vi "driveStop.vi"() -> ()   [LabVIEW 2011]
uses:
  drivetrain/gear_shift_state.ctl
  drivetrain/drivetrain_drive_mode.ctl
  drivetrain/drivetrain_drive_write_thread.ctl
  drivetrain/drivetrain_globals.vi
panel:
  out "x > y?":bool
  in  "settle time":u32=250
  in  "stop deadband":dbl=1.5
  out "Waveform Chart":cluster{"Left":dbl, "Right":dbl}(graph)
  in  "max stop speed":dbl=1.5
  in  "kI":dbl=-0.008
  in  "kP":dbl=-0.1
  # "Old gains:\n\nkP -0.4\nkI -0.005\nmax stop speed 8\nstop deadband 1.5\nsettle time 250"
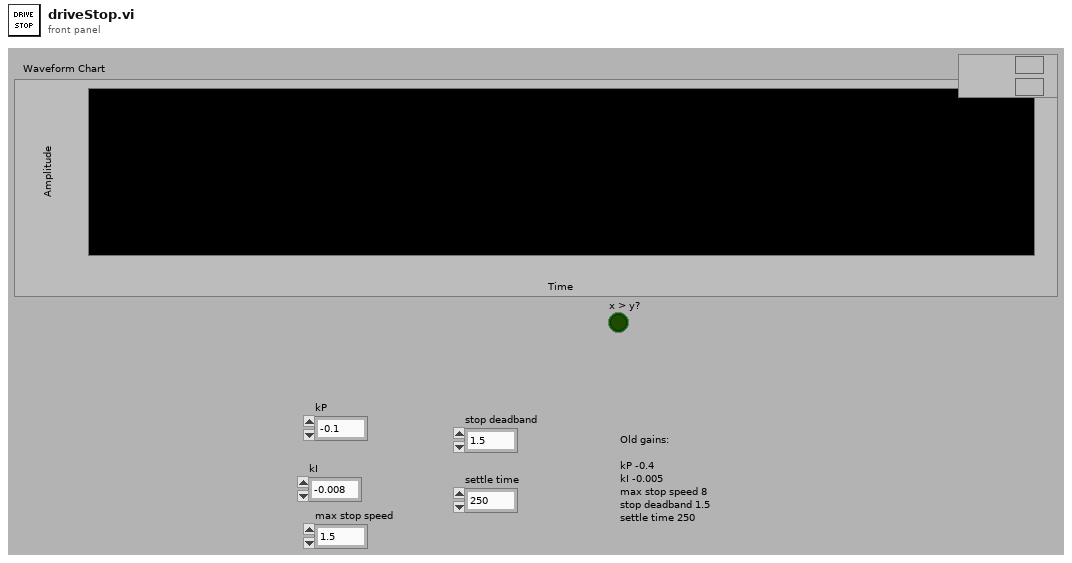
[diagram p1: front panel]
types:
  T1 = typedef "gear_shift_state.ctl" = enum16{"low", "high"}
  T2 = typedef "drivetrain_drive_mode.ctl" = enum16{"open loop", "closed loop"}
  T3 = typedef "drivetrain_drive_write_thread.ctl" = enum16{"Teleop", "Script Engine - Autonomous", "Script Engine - Sequence"}
  T4 = typedef "WPI_RobotDriveDevRef.ctl" = cluster{"DevStatus":errorcluster, "Motors[]":T5[], "Square Inputs":bool, "Max Output":dbl}
  T5 = typedef "WPI_MotorControlDeviceRef.ctl" = cluster{"DeviceStatus":errorcluster, "Type":enum16{"PWM", "CAN"}, "PWM":cluster{"Digital Module":T6, "PWM Channel":T7, "DeadBand":T8}, "CAN":cluster{"Device Number":u8, "Control Mode":T9, "Semaphore":T10, "Max Vout":dbl}, "Invert":bool, "TransformRef":T11, "InvTransformRef":T11}
  T6 = typedef "FPGA_TypedefDigitalModule.ctl" = enum16{"Digital Module 1", "Digital Module 2"}
  T7 = typedef "FPGA_DIOPWMChannel.ctl" = enum8{"PWM 1", "PWM 2", "PWM 3", "PWM 4", "PWM 5", "PWM 6", "PWM 7", "PWM 8", "PWM 9", "PWM 10", "Invalid"}
  T8 = typedef "WPI_PWMDeadband.ctl" = cluster{"Name":string, "maxPositivePwm":i32, "minPositivePwm":i32, "centerPwm":i32, "maxNegativePwm":i32, "minNegativePwm":i32, "angularRange":u16}
  T9 = typedef "WPI_CANJaguar_ControlMode.ctl" = enum8{"Percent VBus", "Current", "Speed", "Position", "Voltage"}
  T10 = typedef "Semaphore RefNum" = refnum<k1>
  T11 = typedef "WPI_PWMTransform_ConPane.ctl" = refnum<vi>
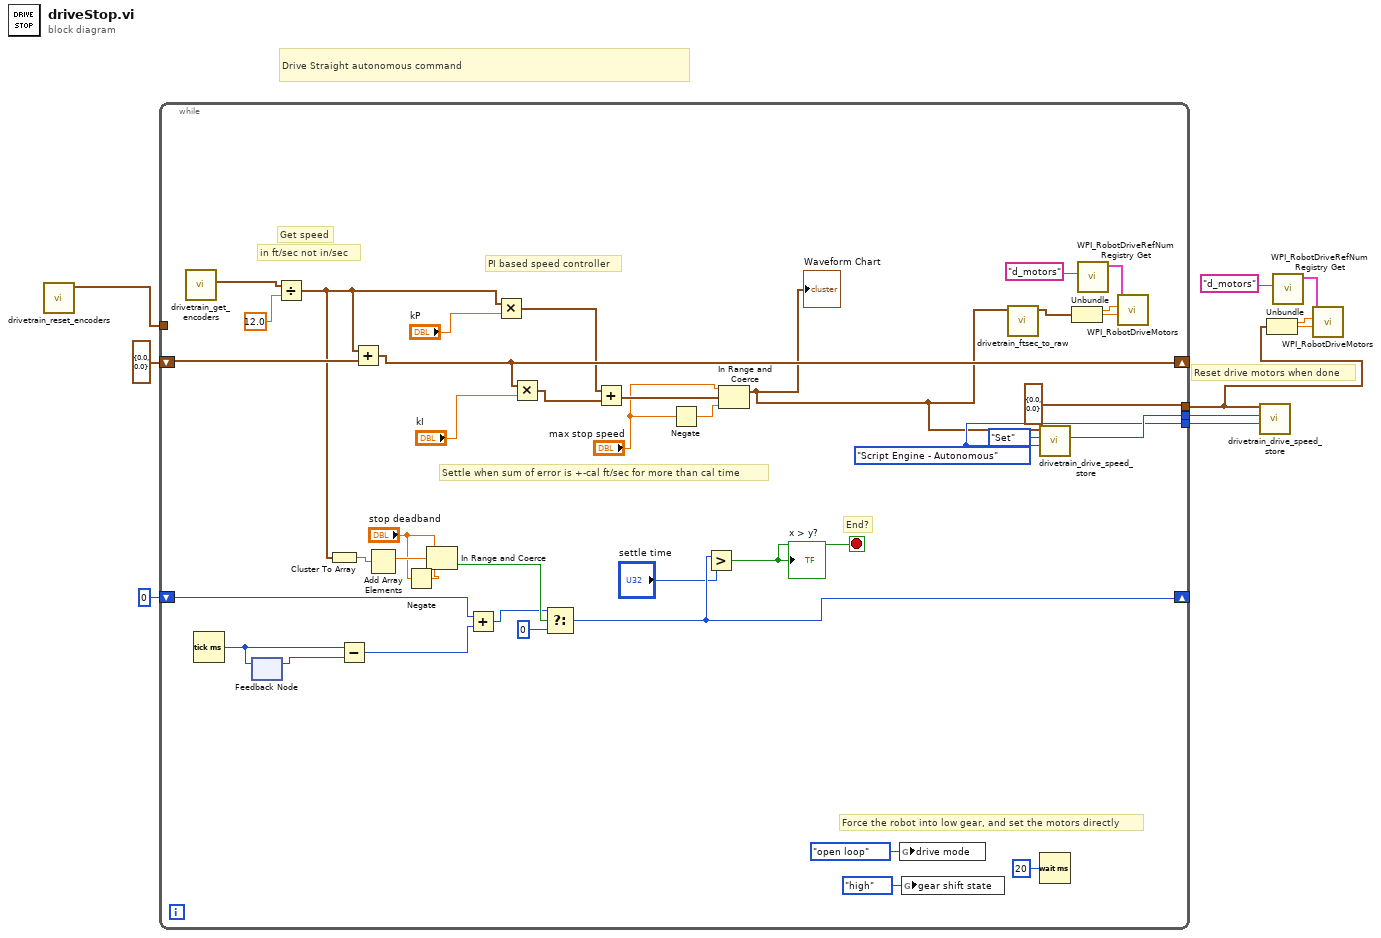
[diagram p0: block diagram]
diagram:
  # "Drive Straight autonomous command"
  # "Reset drive motors when done"
  n1 = call "drivetrain_reset_encoders.vi"() -> ("Distance (in)"=w10:cluster{"Left":dbl, "Right":dbl})  [unwired: 9 in, 2 out]
  n2 = while {
    tunnel: w10 -> [_]
    tunnel: [cluster{"Left":dbl, "Right":dbl} {"Left"=0.0, "Right"=0.0} ("Drive")] -> w5
    tunnel: [w46] -> w9
    tunnel: [w45] -> w8
    shift-right: [w33] -> _
    shift-left: cluster{"Left":dbl, "Right":dbl} {"Left"=0.0, "Right"=0.0} -> [w34]
    shift-right: [w14] -> _
    shift-left: u32 0 -> [w17]
    stop <- w11 stop-if-true
    w45 = drivetrain_drive_write_thread."Script Engine - Autonomous" ("Write Thread")
    w46 = enum16{"Set", "Get"}."Set" ("data_store_mode")
    # "Settle when sum of error is +-cal ft/sec for more than cal time"
    # "PI based speed controller"
    # "in ft/sec not in/sec"
    # "Get speed"
    # "End?"
    # "Force the robot into low gear, and set the motors directly"
    n3 = call "drivetrain_get_encoders.vi"() -> ("Velocity (in/sec)"=w37:cluster{"Left":dbl, "Right":dbl})  [unwired: 9 in, 2 out]
    n4 = Tick Count (ms)() -> (millisecond timer value=w20:u32)
    n5 = feedback-in #1(w20) -> ()
    n6 = feedback #1() -> (w19:u32)  [unwired: 1 in]
    n7 = Divide(x=w37, y=12.0) -> (x/y=w25:cluster{"Left":dbl, "Right":dbl})
    n8 = Cluster To Array(cluster=w25) -> (array=w24:dbl[])
    n9 = Subtract(x=w20, y=w19) -> (x-y=w12:u32)
    n10 = Add(x=w25, y=w34) -> (x+y=w33:cluster{"Left":dbl, "Right":dbl})
    n11 = Add Array Elements(numeric array=w24) -> (sum=w23:dbl)
    n12 = Negate(x="stop deadband") -> (-x=w22:dbl)
    n13 = In Range and Coerce(upper limit="stop deadband", x=w23, lower limit=w22) -> (In Range?=w18:bool)  [unwired: 1 out]
    n14 = Add(x=w17, y=w12) -> (x+y=w16:u32)
    n15 = Multiply(x=w25, y="kP") -> (x*y=w31:cluster{"Left":dbl, "Right":dbl})
    n16 = Multiply(x=w33, y="kI") -> (x*y=w30:cluster{"Left":dbl, "Right":dbl})
    n17 = Select(t=w16, s=w18, f=u32 0) -> (s? t:f=w14:u32)
    n18 = Add(x=w31, y=w30) -> (x+y=w29:cluster{"Left":dbl, "Right":dbl})
    n19 = Negate(x="max stop speed") -> (-x=w28:dbl)
    n20 = Greater?(x=w14, y="settle time") -> (0:w11:bool)
    "x > y?" <- w11
    n21 = In Range and Coerce(upper limit="max stop speed", x=w29, lower limit=w28) -> (coerced(x)=w26:cluster{"Left":dbl, "Right":dbl})  [unwired: 1 out]
    "Waveform Chart" <- w26
    n22 = global write "drivetrain_globals.vi" "drive mode"(drivetrain_drive_mode."open loop" ("drive mode")) -> ()
    n23 = global write "drivetrain_globals.vi" "gear shift state"(gear_shift_state."high" ("gear shift state")) -> ()
    n24 = call "drivetrain_ftsec_to_raw.vi"("Drive Data"=w26) -> ("Drive Data Out"=w38:cluster{"Left":dbl, "Right":dbl})  [unwired: 10 in]
    n25 = call "drivetrain_drive_speed_store.vi"("Write Thread"=w45, "data_store_mode"=w46, "drive data"=w26) -> ()  [unwired: 7 in, 2 out]
    n26 = Wait (ms)(milliseconds to wait=u32 20) -> ()  [unwired: 1 out]
    n27 = Unbundle(w38) -> ("Left"=w40:dbl, "Right"=w41:dbl)
    n28 = call <vilib>:"WPI_RobotDriveRefNum Registry Get.vi"("refnum name"="d_motors") -> ("RobotDriveDevRef"=w43:T4)  [unwired: 9 in, 1 out]
    n29 = call <vilib>:"WPI_RobotDriveMotors.vi"("RightSpeed"=w41, "LeftSpeed"=w40, "RobotDriveDevRef"=w43) -> ()  [unwired: 7 in, 2 out]
  }
  n30 = call "drivetrain_drive_speed_store.vi"("Write Thread"=w8, "data_store_mode"=w9, "drive data"=w5) -> ()  [unwired: 7 in, 2 out]
  n31 = Unbundle(w5) -> ("Left"=w7:dbl, "Right"=w6:dbl)
  n32 = call <vilib>:"WPI_RobotDriveRefNum Registry Get.vi"("refnum name"="d_motors") -> ("RobotDriveDevRef"=w3:T4)  [unwired: 9 in, 1 out]
  n33 = call <vilib>:"WPI_RobotDriveMotors.vi"("RightSpeed"=w6, "LeftSpeed"=w7, "RobotDriveDevRef"=w3) -> ()  [unwired: 7 in, 2 out]
